vi "BBox.vi"() -> ()   [LabVIEW 2025]
panel:
  in  "Python version":u16(ring)=2 items=["3.12", "3.11", "3.10", "3.9", "3.8"]
  in  "Gain":sgl min=-20 max=30 step=0.5 format="%2.1g"
  out "Beam result":bool
  out "AAKit result":bool
  out "Freq result":bool
  out "T/R result":bool
  out "init result":bool
  out "Final state":bool
  in  "TX/RX switch":bool
  in  "Frequency(GHz)":sgl=28.0 min=26.5 max=29.5 step=0.5 format="%#_3f"
  in  "error in (no error)":errorcluster
  in  "Please assign module path (TLKCore_vx.x.x_xxx/main.py)":path=path "C:/TLKCore/main.py"
  in  "Phi":i16 min=0 max=360 step=1 format="%3d"
  in  "Theta":i16 min=0 max=60 step=1 format="%2d"
  out "DR range":sgl[](array[numeric]) caption="Dynamic Range (dB)"
  in  "Please input AAKit Name":string="AAKIT_TMYTEK-4x4_ONE_28_IDEAL"
  out "Current AAKit List":string[](array[string])
  in  "Please assign SN":string="D2230E013-28"
  out "Scanned List (SN,IP,dev_type)":string[](array[string])
  out "Exception message":T1
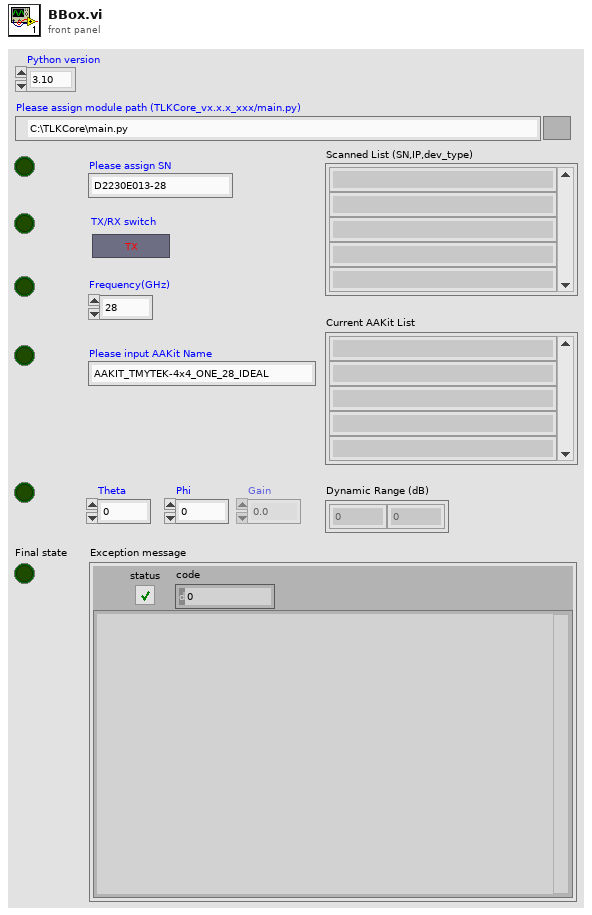
[diagram p1: front panel]
types:
  T1 = cluster{"status":bool, "code":i32, "Exception message":string}
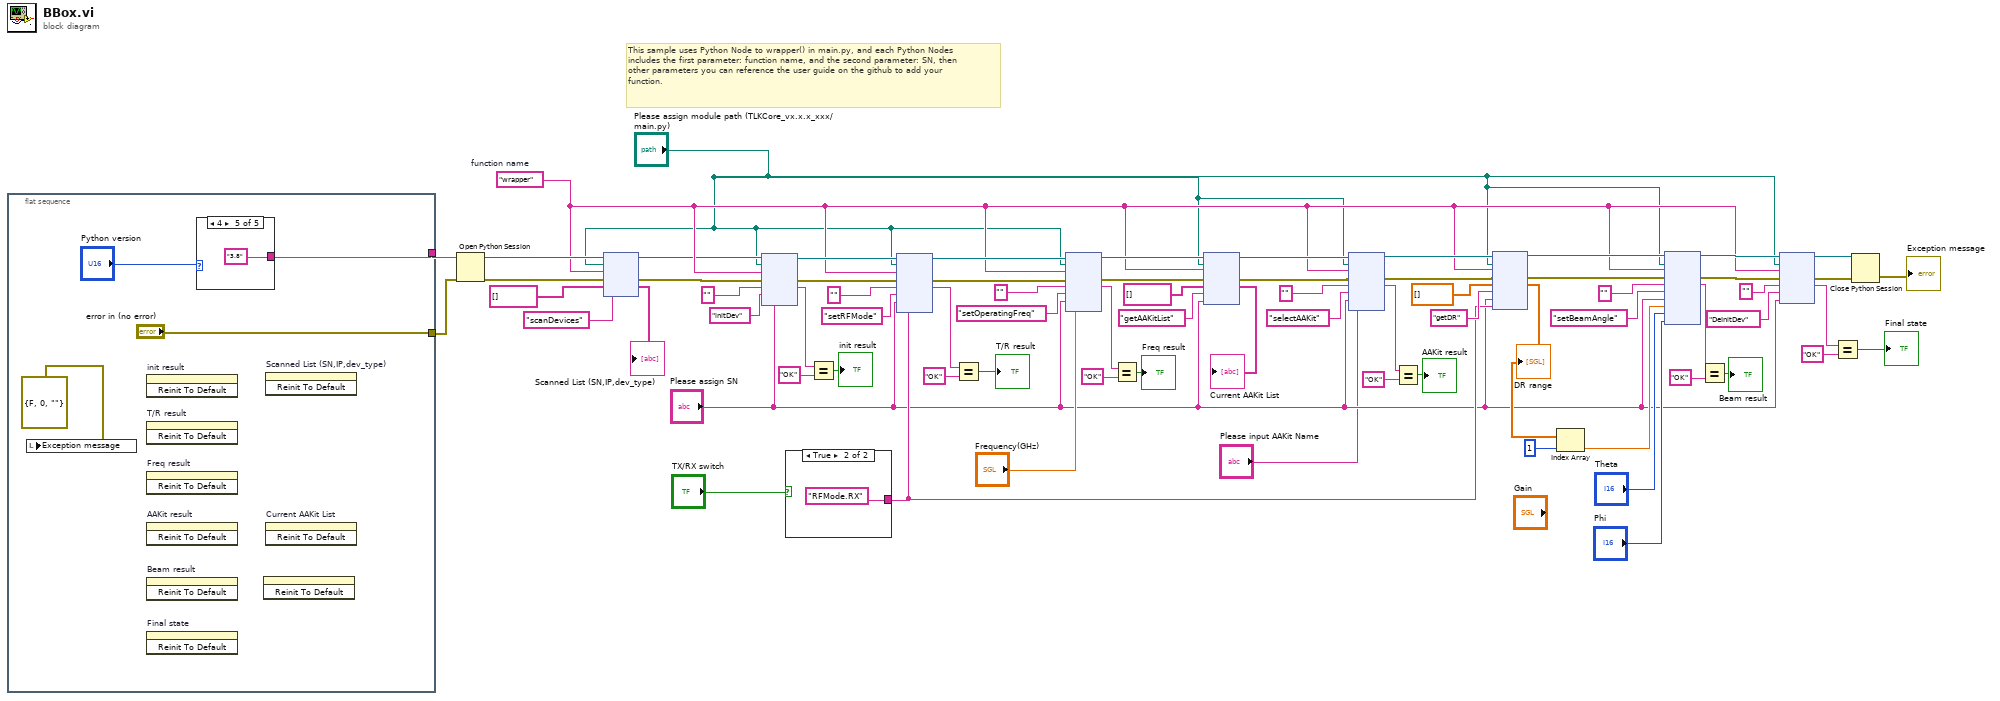
[diagram p0: block diagram]
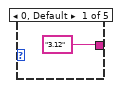
[diagram p2: hidden frame]
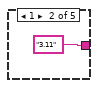
[diagram p3: hidden frame]
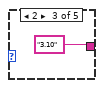
[diagram p4: hidden frame]
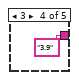
[diagram p5: hidden frame]
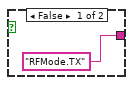
[diagram p6: hidden frame]
diagram:
  w37 = "wrapper"  # function name
  # "This sample uses Python Node to wrapper() in main.py, and each Python Nodes includes the first parameter: function name, and the second parameter: SN, then other parameters you can reference the user guide on the github to add your function."
  n1 = flat-sequence {
    tunnel: ["error in (no error)"] -> w28
    tunnel: [w74] -> w2
    frame #0 {
      n2 = local write "Exception message"(errorcluster {"status"=FALSE, "code"=0, "source"=""} ("Exception message")) -> ()
      n3 = invoke on="init result" class="Bool (strict)" method="Reinit To Default"() -> ()  [unwired: 3 in, 3 out]
      n4 = invoke on="T/R result" class="Bool (strict)" method="Reinit To Default"() -> ()  [unwired: 3 in, 3 out]
      n5 = invoke on="Freq result" class="Bool (strict)" method="Reinit To Default"() -> ()  [unwired: 3 in, 3 out]
      n6 = invoke on="AAKit result" class="Bool (strict)" method="Reinit To Default"() -> ()  [unwired: 3 in, 3 out]
      n7 = invoke on="Beam result" class="Bool (strict)" method="Reinit To Default"() -> ()  [unwired: 3 in, 3 out]
      n8 = invoke on="Final state" class="Bool (strict)" method="Reinit To Default"() -> ()  [unwired: 3 in, 3 out]
      n9 = case shown="4" "Python version" {
        tunnel: ["3.12" ("python version") "3.11" ("python version") "3.10" ("python version") "3.9" ("python version") "3.8" ("python version")] -> w74
        frame 0, Default {
        }
        frame 1 {
        }
        frame 2 {
        }
        frame 3 {
        }
        frame 4 {
        }
      }
      n10 = invoke on="DR range" class="Arr (strict)" method="Reinit To Default"() -> ()  [unwired: 3 in, 3 out]
      n11 = invoke on="Scanned List (SN,IP,dev_type)" class="Arr (strict)" method="Reinit To Default"() -> ()  [unwired: 3 in, 3 out]
      n12 = invoke on="Current AAKit List" class="Arr (strict)" method="Reinit To Default"() -> ()  [unwired: 3 in, 3 out]
    }
  }
  n13 = Open Python Session(python version=w2, 3:w28) -> (session out=w73:refnum<k35>, error out=w1:errorcluster)  [unwired: 1 in]
  n14 = node ("Python Node")(w73, "Please assign module path (TLKCore_vx.x.x_xxx/main.py)", w37, w1, string[] [], "scanDevices") -> (w30:refnum<k35>, w72:errorcluster, →"Scanned List (SN,IP,dev_type)":string[])  [unwired: 1 in, 2 out]
  n15 = node(w30, "Please assign module path (TLKCore_vx.x.x_xxx/main.py)", w37, w72, "", "initDev", "Please assign SN") -> (w63:refnum<k35>, w64:errorcluster, w15:string)  [unwired: 2 in, 2 out]
  n16 = case shown="True" "TX/RX switch" {
    tunnel: ["RFMode.TX" ("RF Mode string") "RFMode.RX" ("RF Mode string")] -> w25
    frame False {
    }
    frame True {
    }
  }
  n17 = Equal?(x=w15, y="OK") -> (x = y?=→"init result":bool)
  n18 = node(w63, "Please assign module path (TLKCore_vx.x.x_xxx/main.py)", w37, w64, "", "setRFMode", "Please assign SN", w25) -> (w56:refnum<k35>, w55:errorcluster, w13:string)  [unwired: 3 in, 2 out]
  n19 = Equal?(x=w13, y="OK") -> (x = y?=→"T/R result":bool)
  n20 = node(w56, "Please assign module path (TLKCore_vx.x.x_xxx/main.py)", w37, w55, "", "setOperatingFreq", "Please assign SN", "Frequency(GHz)") -> (w50:refnum<k35>, w49:errorcluster, w10:string)  [unwired: 3 in, 2 out]
  n21 = Equal?(x=w10, y="OK") -> (x = y?=→"Freq result":bool)
  n22 = node(w50, "Please assign module path (TLKCore_vx.x.x_xxx/main.py)", w37, w49, string[] [], "getAAKitList", "Please assign SN") -> (w47:refnum<k35>, w46:errorcluster, →"Current AAKit List":string[])  [unwired: 2 in, 2 out]
  n23 = node(w47, "Please assign module path (TLKCore_vx.x.x_xxx/main.py)", w37, w46, "", "selectAAKit", "Please assign SN", "Please input AAKit Name") -> (w42:refnum<k35>, w43:errorcluster, w7:string)  [unwired: 3 in, 2 out]
  n24 = Equal?(x=w7, y="OK") -> (x = y?=→"AAKit result":bool)
  n25 = node(w42, "Please assign module path (TLKCore_vx.x.x_xxx/main.py)", w37, w43, sgl[] [], "getDR", "Please assign SN", w25) -> (w41:refnum<k35>, w40:errorcluster, w35:sgl[])  [unwired: 3 in, 2 out]
  "DR range" <- w35
  n26 = Index Array(array=w35, index=1) -> (element=w33:sgl)
  n27 = node(w41, "Please assign module path (TLKCore_vx.x.x_xxx/main.py)", w37, w40, "", "setBeamAngle", "Please assign SN", w33, "Theta", "Phi") -> (w38:refnum<k35>, w39:errorcluster, w4:string)  [unwired: 5 in, 2 out]
  n28 = Equal?(x=w4, y="OK") -> (x = y?=→"Beam result":bool)
  n29 = node(w38, "Please assign module path (TLKCore_vx.x.x_xxx/main.py)", w37, w39, "", "DeInitDev", "Please assign SN") -> (w60:refnum<k35>, w59:errorcluster, w20:string)  [unwired: 2 in, 2 out]
  n30 = Equal?(x=w20, y="OK") -> (x = y?=→"Final state":bool)
  n31 = Close Python Session(session in=w60, error in=w59) -> (11:→"Exception message":errorcluster)
